vi "clearpath_parse_system_status.vi"(0 "ClearpathComm":T1) -> (1 "Data Valid?":bool=TRUE, 2 "Uptime":i32, 3 "Right Motor Current":dbl, 4 "Left Motor Current":dbl, 5 "Controls Current":dbl, 6 "Battery Voltage":dbl)   [LabVIEW 2012, in "clearpath_interface.lvlib"]
doc: "Parses general system status (voltage, current, and temperatures). (Message type 0x8004)"
uses:
  clearpath_interface.lvlib
  cwrap_crio.dll
panel:
  # "System Status Data"
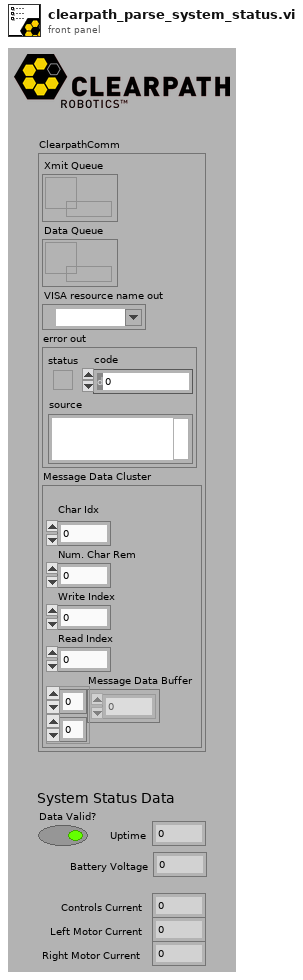
[diagram p1: front panel]
types:
  T1 = cluster{"Xmit Queue":refnum<queue>, "Data Queue":refnum<queue>, "VISA resource name out":refnum<visa-resource-name>, "error out":errorcluster, "Message Data Cluster":cluster{"\nChar Idx":u8, "Num. Char Rem":u8, "Write Index":u8, "Read Index":u8, "Message Data Buffer":u8[][]}}
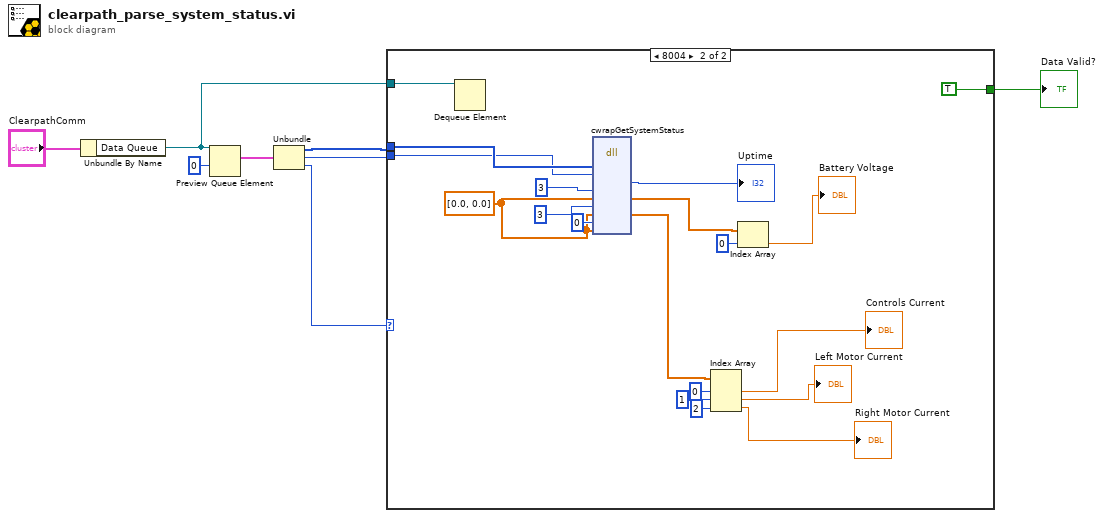
[diagram p0: block diagram]
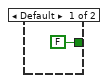
[diagram p2: hidden frame]
diagram:
  n1 = Unbundle By Name("ClearpathComm") -> ("Data Queue"=w1:refnum<queue>)
  n2 = Preview Queue Element(queue=w1, timeout in ms (-1)=0) -> (element=w6:cluster{u8[], "Length":i32, "Type":i32})  [unwired: 1 in, 3 out]
  n3 = Unbundle(w6) -> (w3:u8[], "Length"=w4:i32, "Type"=w5:i32)
  n4 = case shown="8004" w5 {
    tunnel: w4 -> [_ w17]
    tunnel: w3 -> [_ w18]
    tunnel: [FALSE TRUE] -> w2
    tunnel: w1 -> [_ w10]
    frame Default {
    }
    frame 32772 {
      w21 = dbl[] [0.0, 0.0] ("Array")
      n5 = Dequeue Element(queue=w10) -> ()  [unwired: 2 in, 4 out]
      n6 = dll-call lib="C:/Users/cartersm/Documents/GitHub/IGVC-2013/Code/Project 1.0/Motors/Husky/cwrap_cRIO.*" fn="cwrapGetSystemStatus"("packet"=w18, "len"=w17, "voltage_count"=i8 3 ("enc_count"), "voltage"=w21, "current_count"=i8 3, "current"=w21, "temp_count"=i8 0, "temp"=w21) -> ("uptime"=→"Uptime":u32, "voltage"=w26:dbl[], "current"=w22:dbl[])  [unwired: 11 in, 2 out]
      n7 = Index Array(array=w22, index #1=0 ("index"), index #2=1 ("index"), index #3=2 ("index")) -> (element #1=→"Controls Current":dbl, element #2=→"Left Motor Current":dbl, element #3=→"Right Motor Current":dbl)
      n8 = Index Array(array=w26, index=0) -> (element=→"Battery Voltage":dbl)
    }
  }
  "Data Valid?" <- w2
